vi "Sperre thrust alloc Minerva.vi"(0 "Thruster rpms":dbl[](array[numeric]), 1 "manip14":u8, 2 "manip15":u8, 3 "manip16":u8, 5 "error in":errorcluster, 6 "dim 1+2":u8, 7 "Light 1":bool, 8 "dim 3+4":u8, 9 "Light 2":bool, 10 "digital2":u8, 11 "Light 3":bool, 12 "camera":u8=2, 13 "Light 4":bool, 17 "HMI 1":bool, 18 "HMI 2":bool) -> (14 "telebuf":u8[](array[numeric]), 19 "error IO":errorcluster)   [LabVIEW 2014]
uses:
  <vilib>/imath/engines/lvmath2/RunTimeEngine/BuiltInFunctions/uint8/NIMS_uint8(int).vi
  <instcachedir>/0/NIMS_uint8(int)_9D6EF81F86254677BB00410F9E5C6A1D.lvgen/NIMS_uint8(int)_9D6EF81F86254677BB00410F9E5C6A1D_001.vi
  <vilib>/imath/engines/lvmath2/RunTimeEngine/BuiltInFunctions/round/NIMS_round(DBL-S).vi
  <vilib>/imath/engines/lvmath2/RunTimeEngine/BuiltInFunctions/uint8/NIMS_uint8(real).vi
  <instcachedir>/0/NIMS_uint8(real)_CAA419FBB1354DA296C59E18C46DECF0.lvgen/NIMS_uint8(real)_CAA419FBB1354DA296C59E18C46DECF0_000.vi
  <instcachedir>/0/NIMS_uint8(int)_9D6EF81F86254677BB00410F9E5C6A1D.lvgen/NIMS_uint8(int)_9D6EF81F86254677BB00410F9E5C6A1D_000.vi
  <vilib>/imath/engines/lvmath2/RunTimeEngine/IndexReplace/NIMS V(S)=S.vi
  <instcachedir>/0/NIMS V(S)=S_2D52C4EC15D8415E870AEE69FB516CCA.lvgen/NIMS V(S)=S_2D52C4EC15D8415E870AEE69FB516CCA_003.vi
  <vilib>/imathl/engines/lvmath/Functions/Error Handling/Create Error.vi
  <vilib>/imath/engines/lvmath2/RunTimeEngine/BuiltInFunctions/bitand/NIMS_bitand(SorS,SorS).vi
  <instcachedir>/0/NIMS V(S)=S_2D52C4EC15D8415E870AEE69FB516CCA.lvgen/NIMS V(S)=S_2D52C4EC15D8415E870AEE69FB516CCA_000.vi
  <vilib>/imath/engines/lvmath2/RunTimeEngine/ErrorHandling/NIMS_Create Error From Enums.vi
  <vilib>/imath/engines/lvmath2/RunTimeEngine/IndexRead/NIMS V(S).vi
  <instcachedir>/0/NIMS V(S)_0488751826AF41519A22953C041130DC.lvgen/NIMS V(S)_0488751826AF41519A22953C041130DC_000.vi
  <vilib>/imath/engines/lvmath2/RunTimeEngine/BuiltInFunctions/bitset/NIMS_bitset(RS,RS,RS).vi
  <vilib>/imath/engines/lvmath2/RunTimeEngine/BuiltInFunctions/bitget/NIMS_bitget(SorS,SorS).vi
  <vilib>/imath/engines/lvmath2/RunTimeEngine/RangeToken/NIMS_Range_R2 - Integer.vi
  <instcachedir>/0/NIMS_Range_R2 - Integer_2D1304BAF97744E0A293025746CBADFC.lvgen/NIMS_Range_R2 - Integer_2D1304BAF97744E0A293025746CBADFC_000.vi
  <vilib>/imath/engines/lvmath2/RunTimeEngine/CommandStatement/MC_CommandStatement_break.vi
  <vilib>/imath/engines/lvmath2/RunTimeEngine/BuiltInFunctions/double/NIMS_double.vi
  <instcachedir>/0/NIMS_double_34E32F64C2B04A25A042F4CA881A0A41.lvgen/NIMS_double_34E32F64C2B04A25A042F4CA881A0A41_002.vi
  <vilib>/imath/engines/lvmath2/RunTimeEngine/BuiltInFunctions/mod/NIMS_mod_no_size_check.vi
  <instcachedir>/0/NIMS_mod_no_size_check_5393E3382FD241D281EEB71DA286C65B.lvgen/NIMS_mod_no_size_check_5393E3382FD241D281EEB71DA286C65B_001.vi
  <vilib>/imath/engines/lvmath2/RunTimeEngine/NodeEndStatement/NIMS_NodeEndStatement_Output.vi
  <instcachedir>/0/NIMS_NodeEndStatement_Output_53EC0D466D134D7ABD903AC30B43404B.lvgen/NIMS_NodeEndStatement_Output_53EC0D466D134D7ABD903AC30B43404B_011.vi
  <vilib>/imath/engines/lvmath2/RunTimeEngine/ErrorHandling/NIMS_Finalize Error.vi
panel:
  in  "Zoom":bool[](array[boolean])
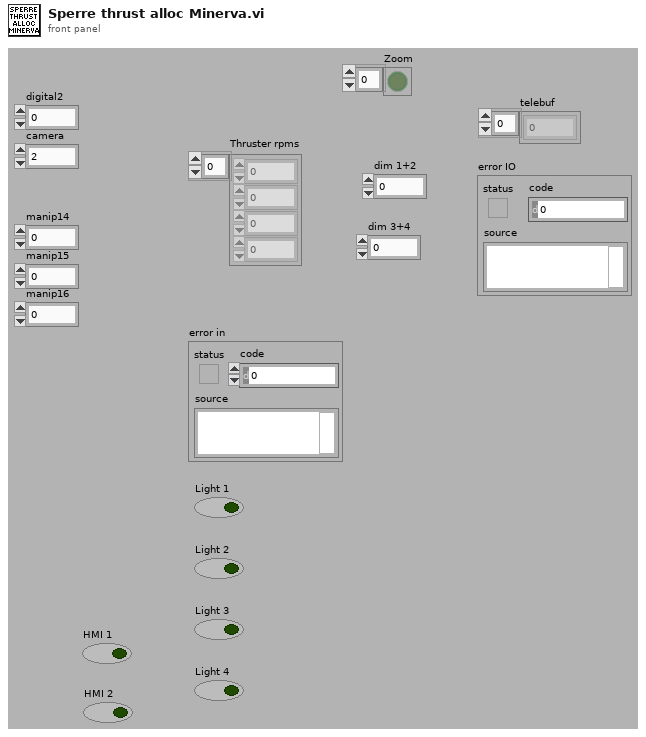
[diagram p1: front panel]
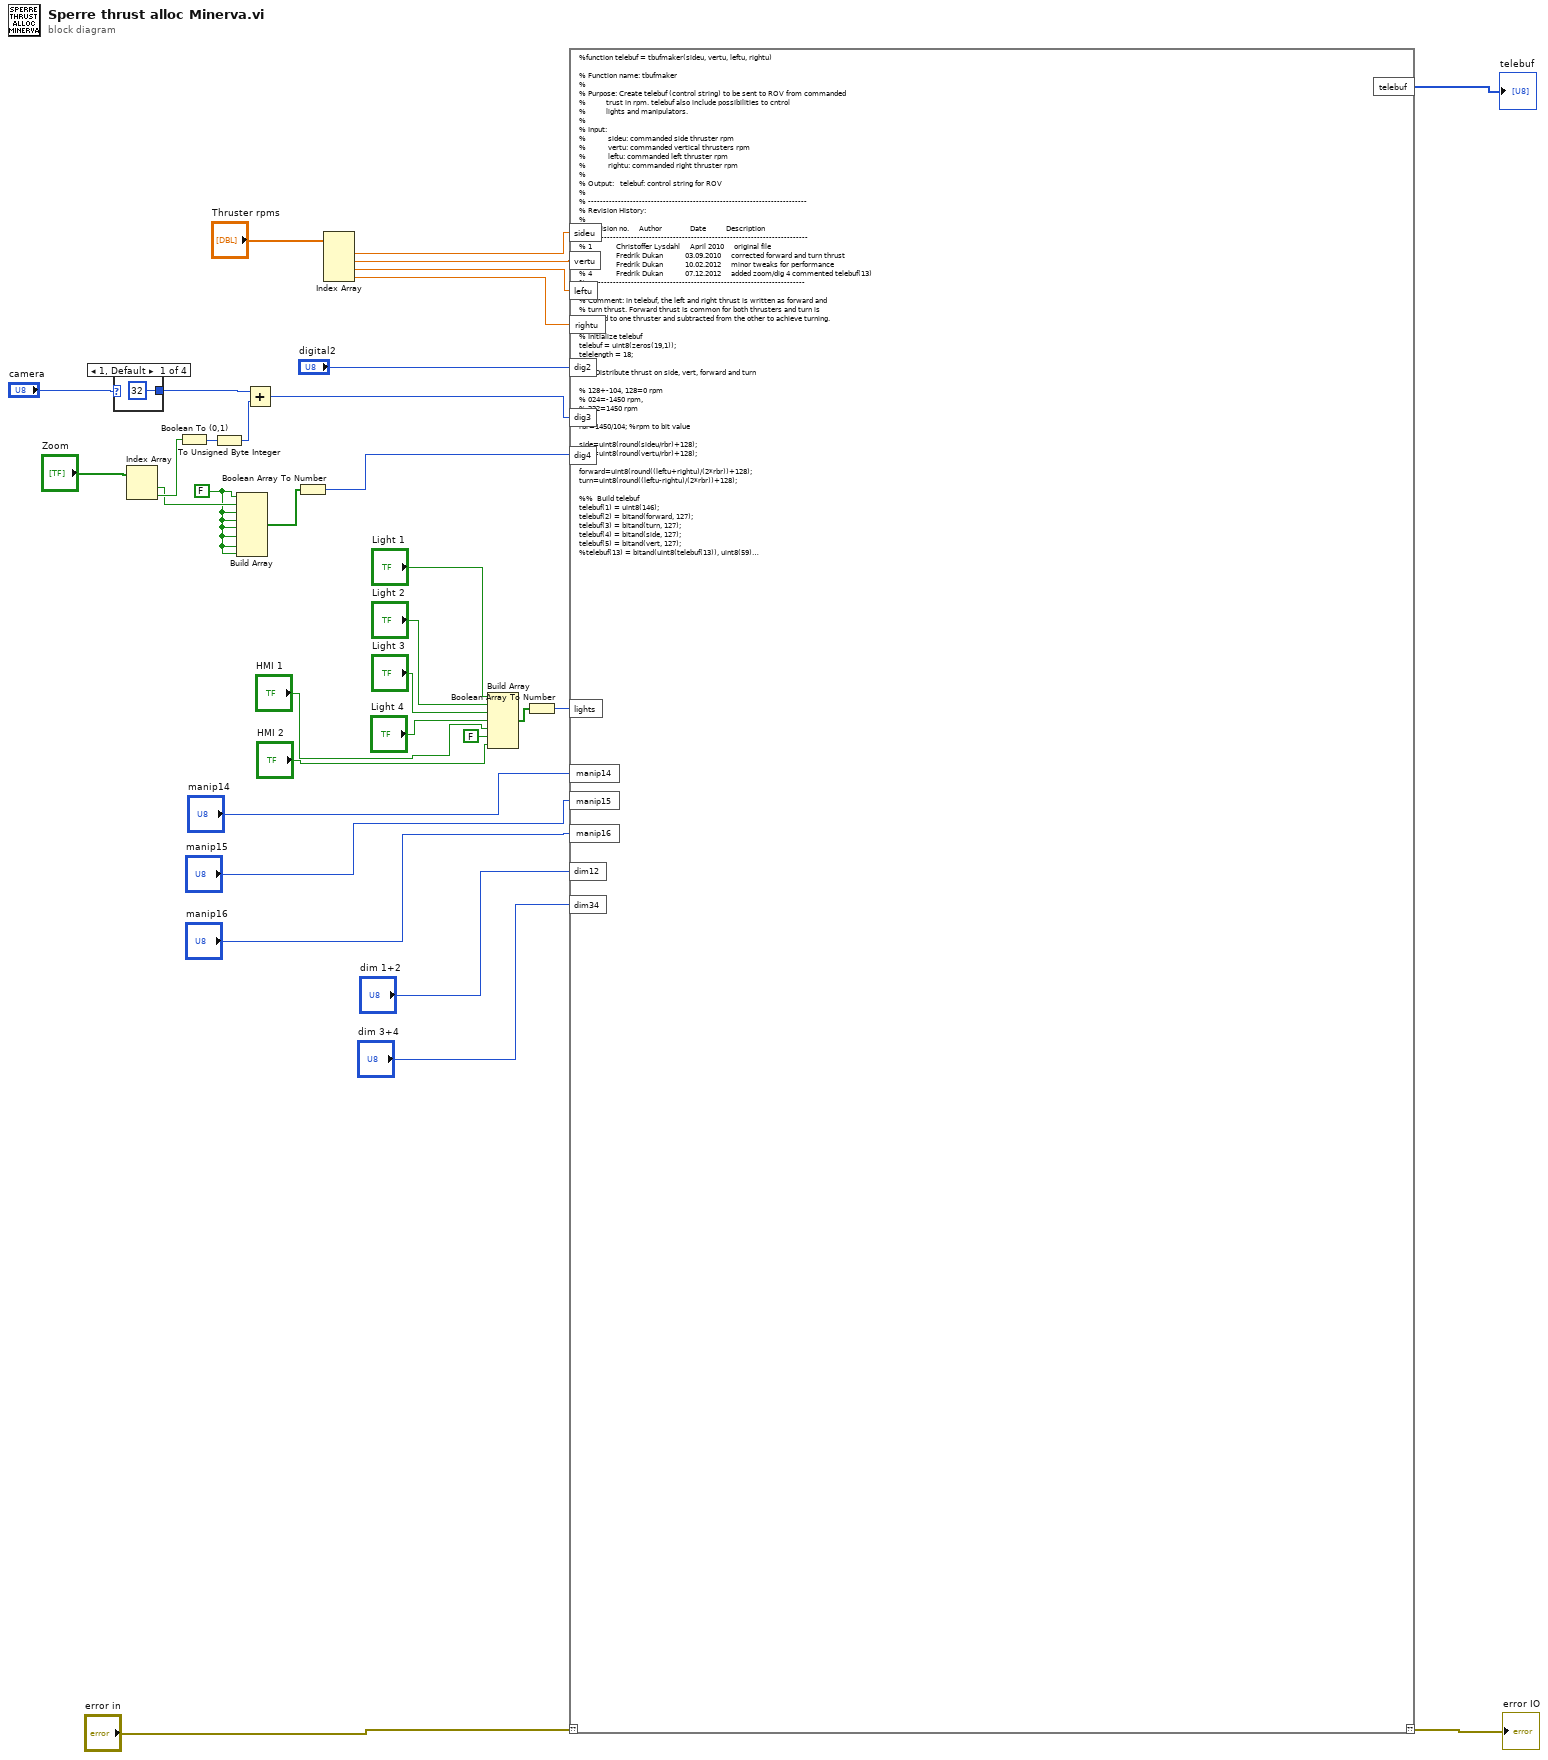
[diagram p0: block diagram]
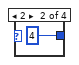
[diagram p2: hidden frame]
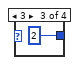
[diagram p3: hidden frame]
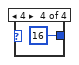
[diagram p4: hidden frame]
diagram:
  w1 = FALSE ("element")
  n1 = case shown="1, Default" "camera" {
    tunnel: [u8 32 u8 4 u8 2 u8 16] -> w9
    frame 1, Default {
    }
    frame 2 {
    }
    frame 3 {
    }
    frame 4 {
    }
  }
  n2 = Index Array(array="Zoom") -> (element #1=w4:bool, element #2=w5:bool)  [unwired: 2 in]
  n3 = Boolean To (0,1)(Boolean=w5) -> (0, 1=w8:i16)
  n4 = To Unsigned Byte Integer(number=w8) -> (unsigned 8bit integer=w7:u8)
  n5 = Build Array(w1, w4, w1, w1, w1, w1, w1, w1) -> (w3:bool[])
  n6 = Add(x=w9, y=w7) -> (x+y=w6:u8)
  n7 = Boolean Array To Number(Boolean array=w3) -> (number=w2:u32)
  n8 = Index Array(array="Thruster rpms") -> (element #1=w22:dbl, element #2=w21:dbl, element #3=w20:dbl, element #4=w19:dbl)  [unwired: 4 in]
  n9 = Build Array("Light 1", "Light 2", "Light 3", "Light 4", "HMI 1", FALSE ("element"), "HMI 2") -> (w31:bool[])
  n10 = Boolean Array To Number(Boolean array=w31) -> (number=w32:u32)
  n11 = mathscript code="%function telebuf = tbufmaker(sideu, vertu, leftu, rightu)\n\n% Function name: tbufmaker\n%\n% Purpose: Create telebuf (control string) to be sent to ROV from commanded\n%          trust in rpm. telebuf also include possibilities to cntrol\n%          lights and manipulators.\n%\n% Input:  \n%           sideu: commanded side thruster rpm\n%           vertu: commanded vertical thrusters rpm\n%           leftu: commanded left thruster rpm\n%           rightu: commanded right thruster rpm\n%\n% Output:   telebuf: control string for ROV\n%\n% -------------------------------------------------------------------------\n% Revision History:\n%\n% Revision no.     Author              Date          Description\n%--------------------------------------------------------------------------\n% 1            Christoffer Lysdahl     April 2010     original file\n% 2            Fredrik Dukan           03.09.2010     corrected forward and turn thrust\n% 3            Fredrik Dukan           10.02.2012     minor tweaks for performance \n% 4            Fredrik Dukan           07.12.2012     added zoom/dig 4 commented telebuf(13)\n%-------------------------------------------------------------------------\n\n% Comment: in telebuf, the left and right thrust is written as forward and\n% turn thrust. Forward thrust is common for both thrusters and turn is \n% added to one thruster and subtracted from the other to achieve turning.\n\n% Initialize telebuf\ntelebuf = uint8(zeros(19,1));\ntelelength = 18;\n\n%% Distribute thrust on side, vert, forward and turn\n\n% 128+-104, 128=0 rpm\n% 024=-1450 rpm,\n% 232=1450 rpm\n\nrbr=1450/104; %rpm to bit value\n\nside=uint8(round(sideu/rbr)+128);\nvert=uint8(round(vertu/rbr)+128);\n\nforward=uint8(round((leftu+rightu)/(2*rbr))+128);\nturn=uint8(round((leftu-rightu)/(2*rbr))+128);\n\n%%  Build telebuf\ntelebuf(1) = uint8(146);\ntelebuf(2) = bitand(forward, 127);\ntelebuf(3) = bitand(turn, 127);\ntelebuf(4) = bitand(side, 127);\ntelebuf(5) = bitand(vert, 127);\n%telebuf(13) = bitand(uint8(telebuf(13)), uint8(59)); %turn off auto heading and depth\ntelebuf(14) = bitset(uint8(telebuf(14)), 7, 0); % note: not needed in matlab\ntelebuf(14) = bitset(uint8(telebuf(14)), 7, bitget(forward, 8));\ntelebuf(14) = bitset(uint8(telebuf(14)), 6, 0); % note: not needed in matlab\ntelebuf(14) = bitset(uint8(telebuf(14)), 6, bitget(turn, 8));\ntelebuf(14) = bitset(uint8(telebuf(14)), 5, 0); % note: not needed in matlab\ntelebuf(14) = bitset(uint8(telebuf(14)), 5, bitget(side, 8));\ntelebuf(14) = bitset(uint8(telebuf(14)), 4, 0); % note: not needed in matlab\ntelebuf(14) = bitset(uint8(telebuf(14)), 4, bitget(vert, 8));\n\n%lights on\ntelebuf(7) = dim12;\ntelebuf(8) = dim34;\ntelebuf(9) = uint8(64);\ntelebuf(10) =lights;\ntelebuf(11) =dig2;\ntelebuf(12) =dig3;\ntelebuf(13) =dig4;\ntelebuf(15) = manip14;\ntelebuf(16) = manip15;\ntelebuf(17) = manip16;\n\n%checksums\nchk = uint8(0);\n\nfor i = 1:telelength - 1\n    chk = chk + telebuf(i);\nend\nchk1 = double(chk);\ncheck1 = bitand(uint8(floor(chk1/256)), 127);\ncheck2 = bitand(mod(chk, 256) , 127);\ntelebuf(18) = check1;\ntelebuf(19) = check2;"("??"="error in", "sideu"=w22, "vertu"=w21, "leftu"=w20, "rightu"=w19, "dim12"="dim 1+2", "dim34"="dim 3+4", "lights"=w32, "manip14"="manip14", "manip15"="manip15", "manip16"="manip16", "dig2"="digital2", "dig3"=w6, "dig4"=w2) -> ("??"=→"error IO":errorcluster, "telebuf"=→"telebuf":u8[])
